vi "555中的放大器.vi"(1 "VCC":dbl, 2 "IN+":dbl, 3 "IN--":dbl, 4 "--VCC":dbl) -> (7 "OUT":dbl)   [LabVIEW 2018]
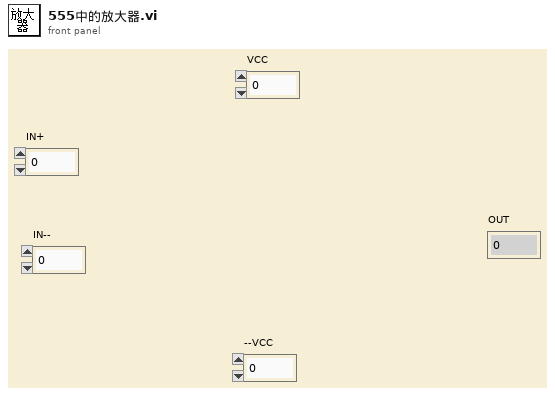
[diagram p1: front panel]
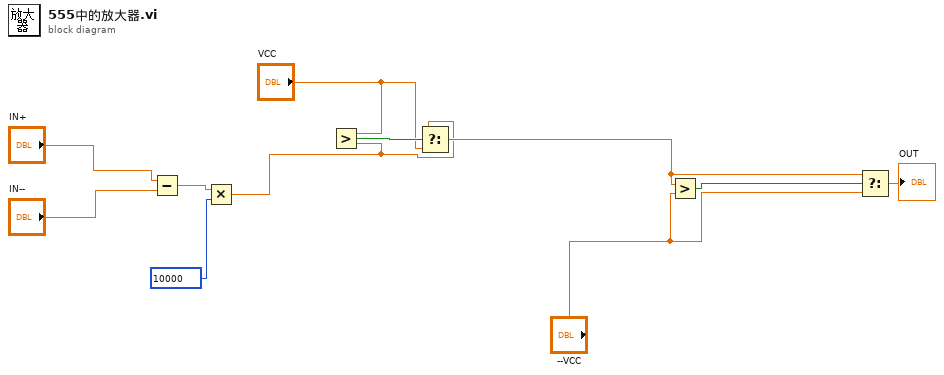
[diagram p0: block diagram]
diagram:
  n1 = Subtract(x="IN+", y="IN--") -> (x-y=w4:dbl)
  n2 = Multiply(x=w4, y=10000) -> (x*y=w1:dbl)
  n3 = Greater?(x="VCC", y=w1) -> (0:w11:bool)
  n4 = Select(t=w1, s=w11, f="VCC") -> (s? t:f=w8:dbl)
  n5 = Greater?(x=w8, y="--VCC") -> (0:w10:bool)
  n6 = Select(t=w8, s=w10, f="--VCC") -> (s? t:f=→"OUT":dbl)
